vi "Open Connection.vi"(0 "Server Address":string, 1 "Authentication":T1, 5 "Port (3306)":u16=3306, 7 "Retries (4)":i32=4, 9 "timeout (15s)":dbl=15.0, 11 "error in (no error)":errorcluster) -> (4 "connection ID out":refnum<k5>, 15 "error out":errorcluster)   [LabVIEW 2014, in "hse-db.lvlib" / "MySQL (TCP).lvlib"]
uses:
  MySQL (TCP).lvlib
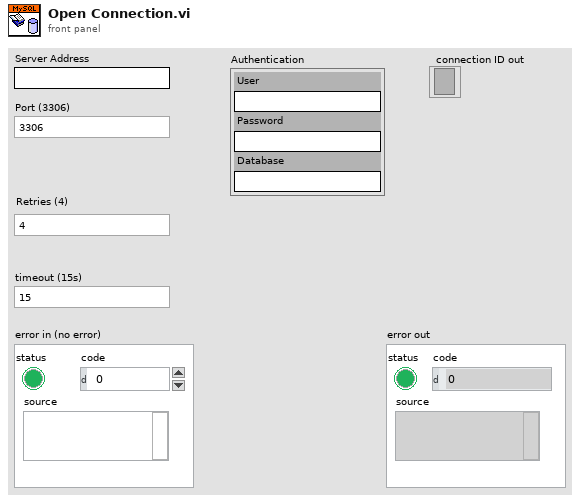
[diagram p1: front panel]
types:
  T1 = cluster{"User":string, "Password":string, "Database":string}
  T2 = typedef "hse-db.lvlib/MySQL (TCP).lvlib/Server Init Data.ctl" = cluster{"Protocol Version":u8, "Server Version":string, "Thread ID":u32, "Scramble Buffer":u8[], "Server Capabilities":u16, "Server Languague":u8, "Server Status":u16}
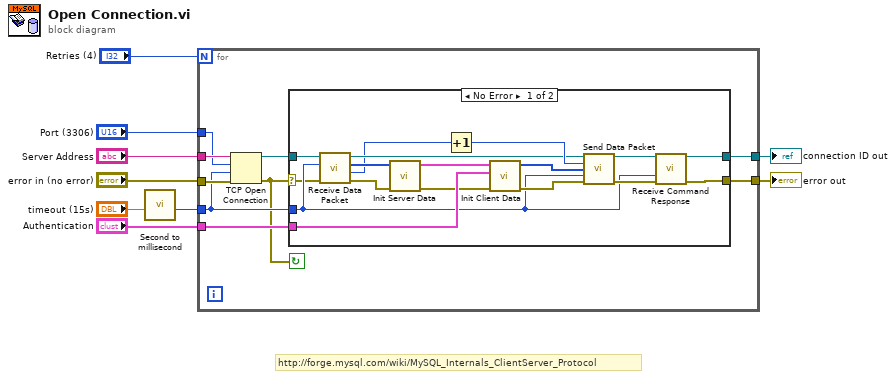
[diagram p0: block diagram]
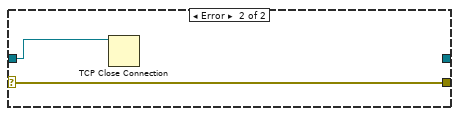
[diagram p2: hidden frame]
diagram:
  # "http://forge.mysql.com/wiki/MySQL_Internals_ClientServer_Protocol"
  n1 = call "Second to millisecond.vi"("Timeout"="timeout (15s)") -> ("Timeout (ms)"=w1:i32)  [unwired: 10 in]
  n2 = for {
    N: "Retries (4)" -> [_]
    tunnel: "Server Address" -> [w18]
    tunnel: "Port (3306)" -> [w17]
    tunnel: "Authentication" -> [w14]
    tunnel: [w12] -> w4
    tunnel: w1 -> [w11]
    tunnel: "error in (no error)" -> [w16]
    tunnel: [w13] -> w5
    stop <- w10 continue-if-true
    n3 = TCP Open Connection(address=w18, remote port or service name=w17, timeout ms (60000)=w11, error in (no error)=w16) -> (connection ID=w15:refnum<k5>, error out=w10:errorcluster)  [unwired: 1 in]
    n4 = case shown="No Error" w10 {
      selector: w10 -> [w19 w37]
      tunnel: w15 -> [w34 w36]
      tunnel: w14 -> [w29 _]
      tunnel: [w24 w37] -> w13
      tunnel: [w22 _] -> w12
      tunnel: w11 -> [w20 _]
      frame No Error {
        n5 = call "Receive Data Packet.vi"("error in"=w19, "Timeout (60000ms)"=w20, "connection ID"=w34) -> ("error out"=w35:errorcluster, "Packet #"=w30:u8, "TCP/IP Data"=w33:u8[], "connection ID out"=w31:refnum<k5>)  [unwired: 5 in]
        n6 = call "Init Server Data.vi"("error in (no error)"=w35, "TCPIP Data"=w33) -> ("error out"=w27:errorcluster, "Server Init Data"=w28:T2)  [unwired: 8 in]
        n7 = Increment(x=w30) -> (x+1=w32:u8)
        n8 = call "Init Client Data.vi"("error in (no error)"=w27, "Authentication"=w29, "Server Init Data"=w28) -> ("error out"=w26:errorcluster, "TCPIP Data"=w25:u8[])  [unwired: 7 in]
        n9 = call "Send Data Packet.vi"("connection ID"=w31, "Packet #"=w32, "TCP/IP Data"=w25, "Timeout (15000ms)"=w20, "error in"=w26) -> ("connection ID out"=w21:refnum<k5>, "error out"=w23:errorcluster)  [unwired: 9 in]
        n10 = call "Receive Command Response.vi"("connection ID"=w21, "Timeout (60000ms)"=w20, "error in (no error)"=w23) -> ("connection ID out"=w22:refnum<k5>, "error out"=w24:errorcluster)  [unwired: 10 in, 1 out]
      }
      frame Error {
        n11 = TCP Close Connection(connection ID=w36) -> ()  [unwired: 2 in, 2 out]
      }
    }
  }
  "error out" <- w5
  "connection ID out" <- w4
